vi "RemoveStep.vi"(8 "error in (no error)":errorcluster, 11 "Project.lvclass In":refnum<class "Project.lvclass">) -> (0 "error out":errorcluster, 2 "StepIdx":i32=-1, 3 "Project.lvclass Out":refnum<class "Project.lvclass">)   [LabVIEW 2014, in "Project.lvclass"]
uses:
  Project.lvclass
  StepSetupDataTypeDefine.ctl
  StepData/Control/AllStepTypeData.ctl
  StepData/Control/StepTypeEnum.ctl
  StepData/Control/MoveData.ctl
  StepData/Control/MeasureData.ctl
  Project.lvclass/Project.ctl
  StepData/StepData.lvclass
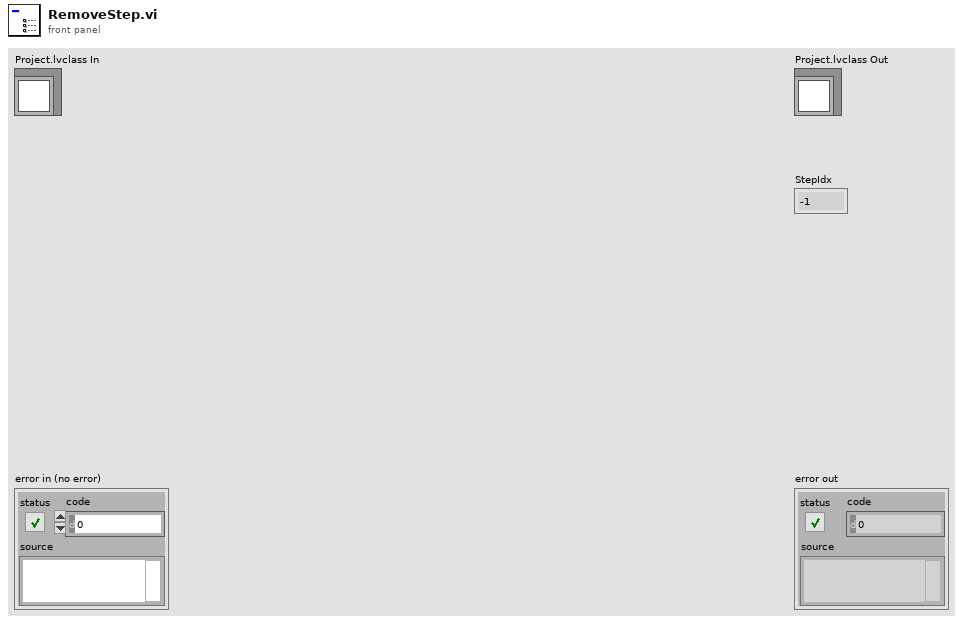
[diagram p1: front panel]
types:
  T1 = typedef "Project.lvclass/StepSetupDataTypeDefine.ctl" = cluster{"AllStepTypeData":T2}[]
  T2 = typedef "StepData.lvclass/AllStepTypeData.ctl" = cluster{"StepName":string, "StepTypeEnum":T3, "MoveData":T4, "MeasureData":T5}
  T3 = typedef "StepData.lvclass/StepTypeEnum.ctl" = enum16{"Move", "Measure"}
  T4 = typedef "StepData.lvclass/MoveData.ctl" = cluster{"Axis":u16, "Position":dbl, "Speed":dbl, "Acc/Dec":dbl, "Mode":u16}
  T5 = typedef "StepData.lvclass/MeasureData.ctl" = cluster{"Sensor No.":i32, "Log?":bool}
  T6 = typedef "Project.lvclass/ProjectDataTableTypeDefine.ctl" = string[][]
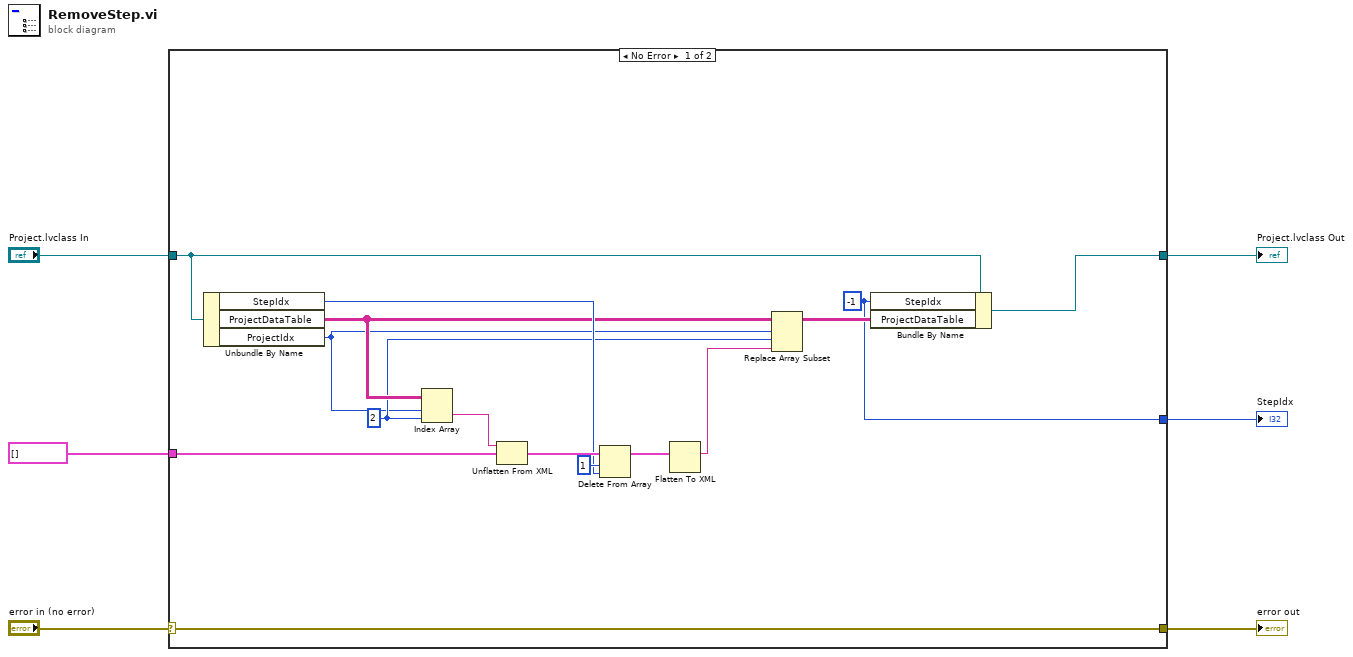
[diagram p0: block diagram]
diagram:
  n1 = case shown="No Error" "error in (no error)" {
    selector: "error in (no error)" -> [w21 w23]
    tunnel: [w21 w23] -> w5
    tunnel: "Project.lvclass In" -> [w20 w22]
    tunnel: [w19 w22] -> w3
    tunnel: T1 [] ("StepSetupClusterArray") -> [w17 _]
    tunnel: [w7 _] -> w1
    frame No Error {
      w7 = -1 ("StepIdx")
      w11 = 2 ("disabled index (col)")
      n2 = Unbundle By Name(w20) -> ("StepIdx"=w14:i32, "ProjectDataTable"=w12:T6, "ProjectIdx"=w10:i32)
      n3 = Index Array(array=w12, index (row)=w10, index (col)=w11) -> (element=w18:string)
      n4 = Unflatten From XML(xml string=w18, type=w17) -> (value=w16:T1)  [unwired: 1 in, 1 out]
      n5 = Delete From Array(array=w16, length=1, index=w14) -> (array with subset deleted=w13:T1)  [unwired: 1 out]
      n6 = Flatten To XML(anything=w13) -> (xml string=w9:string)
      n7 = Replace Array Subset(array=w12, new element=w9, index (row)=w10, index (col)=w11) -> (w8:T6)
      n8 = Bundle By Name(cluster=w20, "StepIdx"=w7, "ProjectDataTable"=w8) -> (w19:refnum<class "Project.lvclass">)
    }
    frame Error {
    }
  }
  "error out" <- w5
  "Project.lvclass Out" <- w3
  "StepIdx" <- w1
